vi "Read Tank Levels.vi"(8 "error in (no error)":errorcluster, 11 "FPGA VI Reference In":T1) -> (0 "error out":errorcluster, 2 "Tanks levels":dbl[](array[numeric]), 3 "FPGA VI Reference Out":T1)   [LabVIEW 2018, in "RT-FPGA Interface API.lvlib"]
uses:
  RT-FPGA Interface API.lvlib
  FPGA ref.ctl
  <vilib>/Utility/error.llb/Error Cluster From Error Code.vi
  <vilib>/rvi/errors/niLvFpgaAdjustHostInterfaceError.vi
  <vilib>/rvi/interface/nirviReadWriteControl/nirviReadWriteControl.xnode
  NiFpgaLv.dll
  <vilib>/rvi/interface/Simulation/niFpgaSimulationCallBeginRW.vi
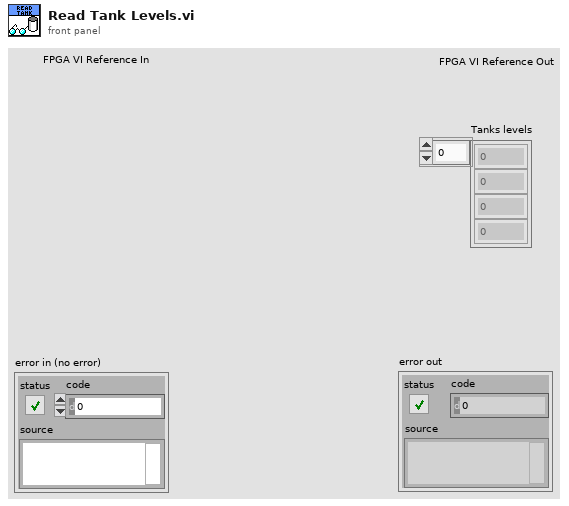
[diagram p1: front panel]
types:
  T1 = typedef "RT-FPGA Interface API.lvlib/FPGA ref.ctl" = refnum<k20>
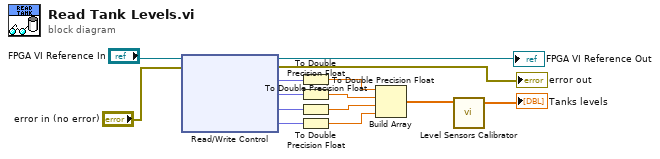
[diagram p0: block diagram]
diagram:
  n1 = xnode "Read/Write Control"("FPGA VI Reference In"="FPGA VI Reference In", "error in"="error in (no error)") -> ("FPGA VI Reference Out"=→"FPGA VI Reference Out":T1, "error out"=→"error out":errorcluster, "Nível Tanque 1"=w14:fxp<+/-,16,5>, "Nível Tanque 2"=w13:fxp<+/-,16,5>, "Nível Tanque 3"=w12:fxp<+/-,16,5>, "Nível Tanque 4"=w11:fxp<+/-,16,5>)
  n2 = To Double Precision Float(number=w14) -> (double precision float=w8:dbl)
  n3 = To Double Precision Float(number=w13) -> (double precision float=w7:dbl)
  n4 = To Double Precision Float(number=w12) -> (double precision float=w6:dbl)
  n5 = To Double Precision Float(number=w11) -> (double precision float=w5:dbl)
  n6 = Build Array(w8, w7, w6, w5) -> (w1:dbl[])
  n7 = call "Level Sensors Calibrator.vi"("Data in"=w1) -> ("Data out"=→"Tanks levels":dbl[])  [unwired: 4 in]
